vi "V_to_I16_USB7855R.vi"(7 "Calibration Constant":cluster{"LSB Weight":u32, "Offset":i32}, 8 "Max/Min Value [V]":dbl, 11 "Input":dbl[](array[numeric])=[0.0, 0.0]) -> (2 "16bit integer":i16[](array[numeric]))   [LabVIEW 2023]
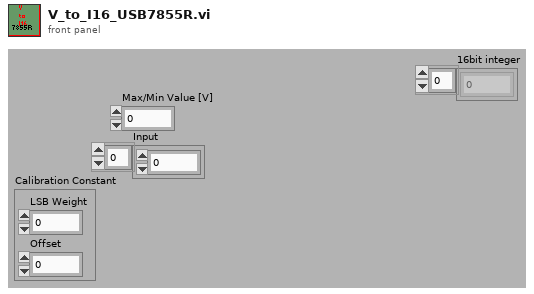
[diagram p1: front panel]
types:
  T1 = enum16{"USB 7855 (AI)", "USB 7855 (AO)", "USB 7855 OEM (AI)", "USB 7855 OEM (AO)", "USB 7856  (AI)", "USB 7856 (AO)", "USB 7856 OEM (AI)", "USB 7856 OEM (AO)"}
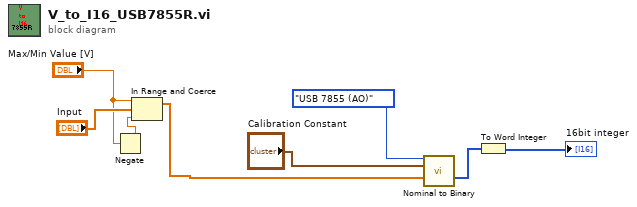
[diagram p0: block diagram]
diagram:
  n1 = Negate(x="Max/Min Value [V]") -> (-x=w6:dbl)
  n2 = In Range and Coerce(upper limit="Max/Min Value [V]", x="Input", lower limit=w6) -> (coerced(x)=w2:dbl[])  [unwired: 1 out]
  n3 = call "Nominal to Binary.vi"("Target Type"=T1."USB 7855 (AO)", "Calibration"="Calibration Constant", "Nominal Value"=w2) -> ("Binary Value"=w5:i32[])  [unwired: 12 in]
  n4 = To Word Integer(number=w5) -> (16bit integer=→"16bit integer":i16[])
